vi "Set Routing and Faulting Custom Device.vi"(8 "error in (no error)":errorcluster, 11 "RAF Custom Device in":refnum<k24>) -> (0 "error out":errorcluster, 3 "RAF Custom Device out":refnum<k24>)   [LabVIEW 2017]
uses:
  NationalInstruments.VeriStand.SystemDefinitionAPI
  Shared/Constants.vi
  <vilib>/NI VeriStand/Custom Device API/Custom Device API.lvlib
  Shared/Switch Shared.lvlib
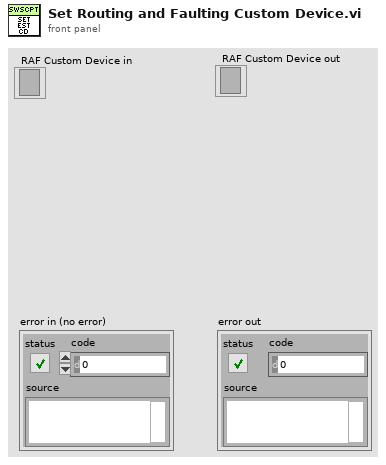
[diagram p1: front panel]
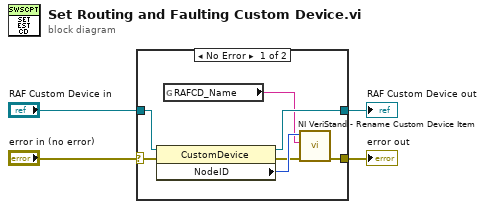
[diagram p0: block diagram]
diagram:
  n1 = case shown="No Error" "error in (no error)" {
    selector: "error in (no error)" -> [w10 w13]
    tunnel: [w6 w13] -> w4
    tunnel: [w11 w12] -> w3
    tunnel: "RAF Custom Device in" -> [w9 w12]
    frame No Error {
      n2 = property class="CustomDevice"(reference=w9, error in=w10) -> (reference out=w11:refnum<k24>, error out=w7:errorcluster, "NodeID"=w8:u64)
      n3 = global read "Constants.vi" "RAFCD_Name"() -> (w5:string)
      n4 = call <vilib>:"NI VeriStand - Rename Custom Device Item.vi"("error in (no error)"=w7, "New Name"=w5, "Item Ref in"=w8) -> ("error out"=w6:errorcluster)  [unwired: 6 in, 2 out]
    }
    frame Error {
    }
  }
  "error out" <- w4
  "RAF Custom Device out" <- w3
